vi "Information.vi"(8 "error in (no error)":errorcluster, 9 "Context":T1, 10 "Information":refnum<class "Information.lvclass">, 11 "Spectrum Recorder too in":refnum<class "Spectrum Recorder too.lvclass">) -> (0 "error out":errorcluster, 3 "Spectrum Recorder too out":refnum<class "Spectrum Recorder too.lvclass">)   [LabVIEW 2021, in "Spectrum Recorder too.lvclass"]
uses:
  Spectrum Recorder too.lvclass
  C:/GitHub/LabActor/Template Module/Template Module.lvclass
  Publish-Subscribe/Interfaces/Information/Information.lvclass
  Publish-Subscribe/Context.ctl
  NHMFL_Core/Libraries/Instruments/Results/Acquired Result/Acquired Result.lvclass
  NHMFL_Core/Libraries/Instruments/Results/Acquired Result/Acquired Result.lvclass/Acquired Result.ctl
  Template Module/Template Module.lvclass/Template Module.ctl
  NHMFL_Core/Libraries/Instruments/Results/Acquired Result/Write Group.vi
  Template Module/Read Logger.vi
  Template Module/Write Logger.vi
  Loggers/Logger/Logger.lvclass
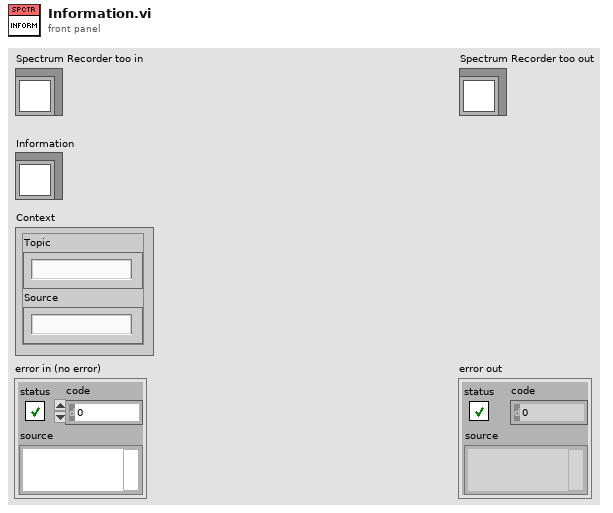
[diagram p1: front panel]
types:
  T1 = typedef "Context.ctl" = cluster{"Topic":string, "Source":string}
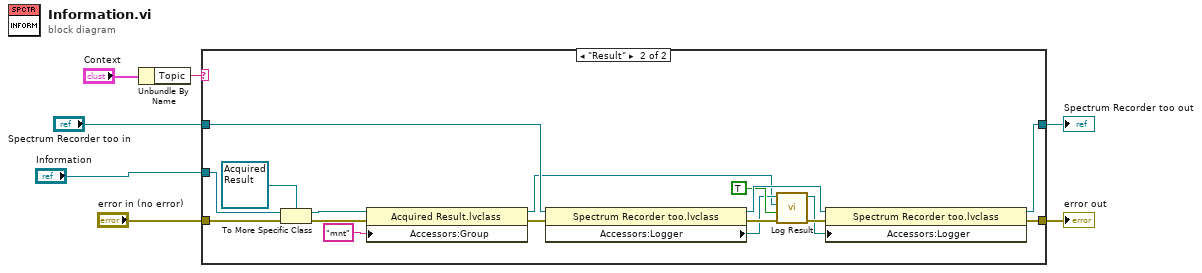
[diagram p0: block diagram]
diagram:
  n1 = Unbundle By Name("Context") -> ("Topic"=w5:string)
  n2 = case shown="\"Result\"" w5 {
    tunnel: "Information" -> [_ w25]
    tunnel: "error in (no error)" -> [w8 w22]
    tunnel: "Spectrum Recorder too in" -> [w9 w15]
    tunnel: [w9 w12] -> w2
    tunnel: [w8 w11] -> w1
    frame "", Default {
    }
    frame "Result" {
      n3 = To More Specific Class(target class=refnum<class "Acquired Result.lvclass"> refnum ("Acquired Result.lvclass"), reference=w25, error in=w22) -> (specific class reference=w10:refnum<class "Acquired Result.lvclass">, error out=w23:errorcluster)
      n4 = property class="Acquired Result.lvclass"(reference=w10, error in=w23, "Accessors:Group"="mnt" ("Group")) -> (reference out=w13:refnum<class "Acquired Result.lvclass">, error out=w14:errorcluster)
      n5 = property class="Spectrum Recorder too.lvclass"(reference=w15, error in=w14) -> (reference out=w21:refnum<class "Spectrum Recorder too.lvclass">, error out=w17:errorcluster, "Accessors:Logger"=w16:refnum<class "Logger.lvclass">)
      n6 = call-dynamic "Log Result.vi"("error in (no error)"=w17, "Timestamp data points"=TRUE, "Result"=w13, "Logger in"=w16) -> ("error out"=w20:errorcluster, "Logger out"=w19:refnum<class "Logger.lvclass">)  [unwired: 6 in]
      n7 = property class="Spectrum Recorder too.lvclass"(reference=w21, error in=w20, "Accessors:Logger"=w19) -> (reference out=w12:refnum<class "Spectrum Recorder too.lvclass">, error out=w11:errorcluster)
    }
  }
  "error out" <- w1
  "Spectrum Recorder too out" <- w2
